vi "sio read.vi"(8 "len":i32, 9 "buf":i8[](array[numeric]), 10 "port":i32) -> (0 "len":i32, 1 "buf out":i8[](array[numeric]), 2 "Status":i32, 3 "port":i32)   [LabVIEW 2015, in "PCOMM.lvlib"]
doc: "int WINAPI sio_read(int port, char *buf, int len);"
uses:
  PCOMM.lvlib
  PCOMM.DLL
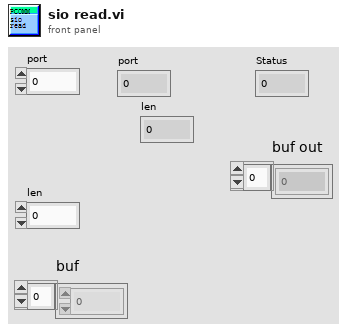
[diagram p1: front panel]
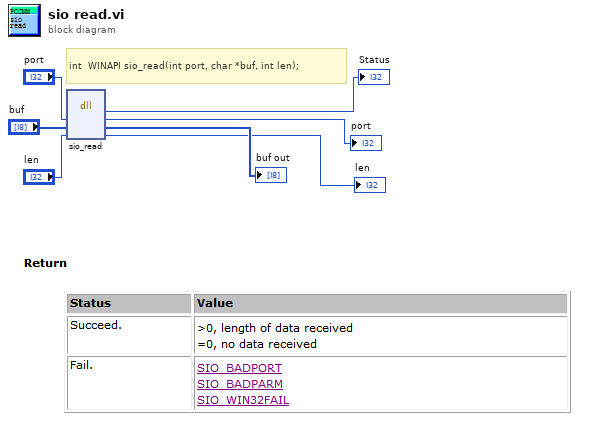
[diagram p0: block diagram]
diagram:
  # "int  WINAPI sio_read(int port, char *buf, int len);"
  n1 = dll-call lib="PTH2Yabs EDesktopLabview串口助手串口助手2.0Ing10_v3.2.0libpcommPCOMM.*" fn="sio_read"("port"="port", "buf"="buf", "len"="len") -> ("返回类型"=→"Status":i32, "port"=→"port":i32, "buf"=→"buf out":i8[], "len"=→"len":i32)  [unwired: 3 in, 2 out]
